vi "compress_alarms_1.vi"(6 "N alr":i32, 7 "table":string, 9 "ALRNames":refnum<data-value>, 10 "Alr_state":T1, 11 "date/time string":string) -> (3 "parameters":string)   [LabVIEW 2019, in "PostgreSQL.lvlib"]
uses:
  PostgreSQL.lvlib
  Alarms/Ctl/ALRs_State.ctl
  Alarms/Alarms.lvlib
panel:
  in  "defaults":string="INSERT INTO public.\"XX00.XX00.XX00.XX00.XX00_FZ.7001\"\n (\"time\", \"on\", \"block\", \"alrname\") \nVALUES ('2017-11-07 12:04:06.000', 'f', 'f', '00000000010000000002000000000300000000040000000005000000000600000000070000000008000000000901234');"
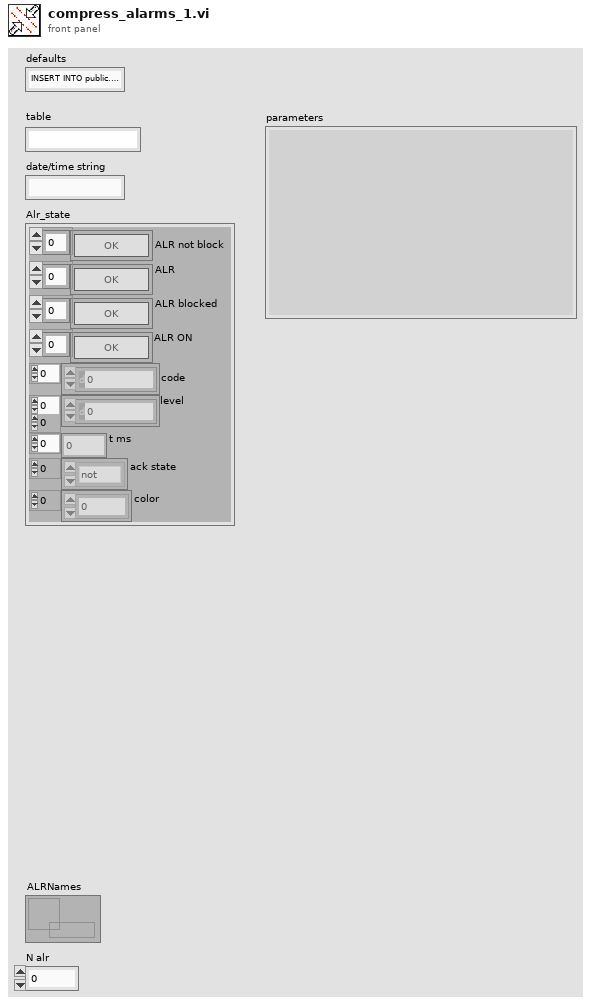
[diagram p1: front panel]
types:
  T1 = typedef "Alarms.lvlib/ALRs_State.ctl" = cluster{"ALR not block":bool[], "ALR":bool[], "ALR blocked":bool[], "ALR ON":bool[], "code":i32[], "level":i32[][], "t ms":u32[], "ack state":enum32{"not", "tripped", "reset", "ack"}[], "color":u32[]}
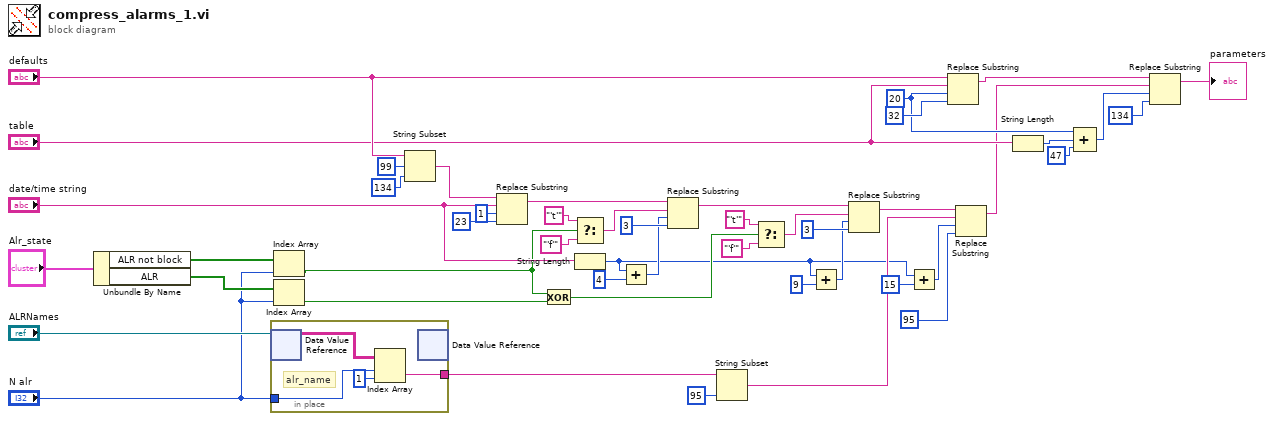
[diagram p0: block diagram]
diagram:
  w36 = 20 ("offset (0)")
  n1 = Unbundle By Name("Alr_state") -> ("ALR not block"=w3:bool[], "ALR"=w14:bool[])
  n2 = in-place {
    in-place-border: "N alr" -> [w51]
    in-place-border: [w50] -> w15
    # "alr_name"
    n3 = in-place-dvr #1("ALRNames") -> (w48:string[][])  [unwired: 1 out]
    n4 = Index Array(array=w48, index (row)=w51, index (col)=1 ("disabled index (col)")) -> (element=w50:string)
    n5 = in-place-dvr #1() -> ()  [unwired: 1 in, 2 out]
  }
  n6 = Index Array(array=w3, index="N alr") -> (element=w1:bool)
  n7 = Index Array(array=w14, index="N alr") -> (element=w16:bool)
  n8 = String Subset(string="defaults", offset (0)=99, length (rest)=134 ("length (rest)")) -> (substring=w37:string)
  n9 = Replace Substring(2:23 ("length (len. of substring)"), 3:1 ("offset (0)"), 4:"date/time string", 5:w37) -> (1:w19:string)  [unwired: 1 out]
  n10 = Exclusive Or(1:w16, 2:w1) -> (0:w27:bool)
  n11 = Select(t="'t'", s=w1, f="'f'") -> (s? t:f=w22:string)
  n12 = String Length(string="date/time string") -> (length=w7:i32)
  n13 = Add(x=w7, y=4) -> (x+y=w11:i32)
  n14 = Replace Substring(2:3 ("x+y"), 3:w11, 4:w22, 5:w19) -> (1:w20:string)  [unwired: 1 out]
  n15 = String Subset(string=w15, length (rest)=95 ("length (rest)")) -> (substring=w26:string)  [unwired: 1 in]
  n16 = Select(t="'t'", s=w27, f="'f'") -> (s? t:f=w31:string)
  n17 = Add(x=w7, y=9) -> (x+y=w9:i32)
  n18 = Replace Substring(2:3 ("x+y"), 3:w9, 4:w31, 5:w20) -> (1:w28:string)  [unwired: 1 out]
  n19 = Add(x=w7, y=15) -> (x+y=w8:i32)
  n20 = Replace Substring(2:32 ("length (len. of substring)"), 3:w36, 4:"table", 5:"defaults") -> (1:w35:string)  [unwired: 1 out]
  n21 = Replace Substring(2:95 ("x+y"), 3:w8, 4:w26, 5:w28) -> (1:w29:string)  [unwired: 1 out]
  n22 = String Length(string="table") -> (length=w43:i32)
  n23 = Compound Arithmetic op=ADD(w36, w43, 47 ("value")) -> (w42:i32)
  n24 = Replace Substring(2:134 ("length (len. of substring)"), 3:w42, 4:w29, 5:w35) -> (1:→"parameters":string)  [unwired: 1 out]
